vi "TemplateModule.GetBroadcasts.vi"(11 "TemplateModule in":refnum<class "TemplateModule.lvclass">) -> (2 "TemplateModule":cluster{"Broadcasts":T1, "Broadcasts":T2}, 3 "TemplateModule out":refnum<class "TemplateModule.lvclass">)   [LabVIEW 2024, in "TemplateModule.lvclass"]
uses:
  TemplateModule.lvclass
  TemplateModule.lvclass/TemplateModule.ctl
  JQMHCore/Module/RQMHModule.lvclass
  C:/Github/JQMH/JQMHCore/Module/RQMHModule.lvclass
  C:/Github/JQMH/Scripting/templates/TemplateModule/TemplateModule.lvclass
  JQMHCore/Shared/Died.ctl
  JQMHCore/Shared/JQMHShared.lvlib
  JQMHCore/Module/StandardBroadcasts.ctl
  Stopped.ctl
  Broadcast Events--cluster.ctl
  JQMHCore/Module/Started.ctl
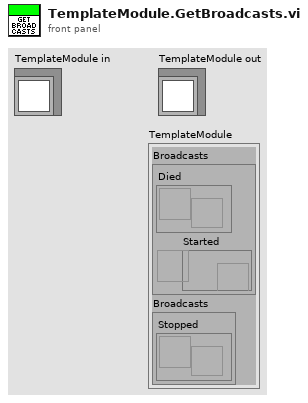
[diagram p1: front panel]
types:
  T1 = typedef "RQMHModule.lvclass/StandardBroadcasts.ctl" = cluster{"Died":refnum<user-event>, "Started":refnum<user-event>}
  T2 = typedef "TemplateModule.lvclass/Broadcast Events--cluster.ctl" = cluster{"Stopped":refnum<user-event>}
  T3 = typedef "TemplateModule.lvclass/Broadcast Events--cluster.ctl" = cluster{"Stopped":refnum<user-event>, "NewControl258813080":refnum<user-event>, "NewControl260354259":refnum<user-event>}
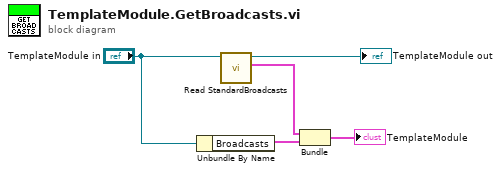
[diagram p0: block diagram]
diagram:
  n1 = Unbundle By Name("TemplateModule in") -> ("Broadcasts"=w5:T3)
  n2 = call "Read StandardBroadcasts.vi"("JQMHCore in"="TemplateModule in") -> ("Broadcasts"=w4:T1, "JQMHCore out"=→"TemplateModule out":refnum<class "TemplateModule.lvclass">)  [unwired: 8 in, 1 out]
  n3 = Bundle("Broadcasts"=w4, "Broadcasts"=w5) -> (→"TemplateModule":cluster{"Broadcasts":T1, "Broadcasts":T3})  [unwired: 1 in]
